vi "JV SN1.vi"(10 "Bool Refnum":refnum<vi>, 11 "Digital in":refnum<vi>) -> ()   [LabVIEW 2018]
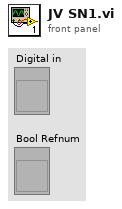
[diagram p1: front panel]
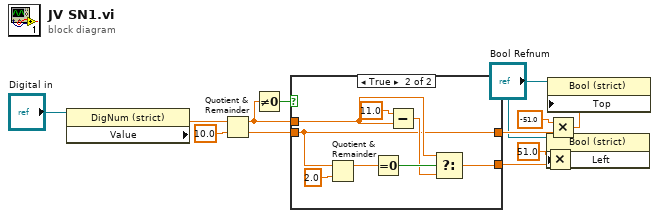
[diagram p0: block diagram]
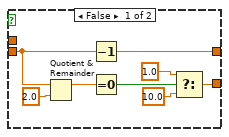
[diagram p2: hidden frame]
diagram:
  n1 = property class="DigNum (strict)"(reference="Digital in") -> ("Value"=w4:dbl)  [unwired: 1 in, 2 out]
  n2 = Quotient & Remainder(x=w4, y=10.0) -> (x-y*floor(x/y)=w6:dbl, floor(x/y)=w5:dbl)
  n3 = Not Equal To 0?(x=w6) -> (x != 0?=w7:bool)
  n4 = case shown="True" w7 {
    tunnel: [w15 w23] -> w13
    tunnel: w6 -> [_ w24]
    tunnel: w5 -> [w16 w23]
    tunnel: [w14 w22] -> w8
    frame False {
      n5 = Quotient & Remainder(x=w16, y=2.0) -> (x-y*floor(x/y)=w20:dbl)  [unwired: 1 out]
      n6 = Decrement(x=w16) -> (x-1=w15:dbl)
      n7 = Equal To 0?(x=w20) -> (x = 0?=w19:bool)
      n8 = Select(t=1.0, s=w19, f=10.0) -> (s? t:f=w14:dbl)
    }
    frame True {
      n9 = Quotient & Remainder(x=w23, y=2.0) -> (x-y*floor(x/y)=w25:dbl)  [unwired: 1 out]
      n10 = Equal To 0?(x=w25) -> (x = 0?=w28:bool)
      n11 = Subtract(x=11.0, y=w24) -> (x-y=w26:dbl)
      n12 = Select(t=w24, s=w28, f=w26) -> (s? t:f=w22:dbl)
    }
  }
  n13 = Multiply(x=51.0, y=w8) -> (x*y=w10:dbl)
  n14 = property on="Property Node" class="Bool (strict)"(reference="Bool Refnum", "Left"=w10) -> ()  [unwired: 1 in, 2 out]
  n15 = Multiply(x=-51.0, y=w13) -> (x*y=w12:dbl)
  n16 = property on="Property Node" class="Bool (strict)"(reference="Bool Refnum", "Top"=w12) -> ()  [unwired: 1 in, 2 out]
